vi "Get-module-path.vi"(8 "error in (no error)":errorcluster, 10 "Module type":T1=enum."Server", 11 "ModComm in":T2) -> (0 "error out":errorcluster, 2 "Module path":path, 3 "ModComm out":T2)   [LabVIEW 2013, in "SLMServer.lvlib" / "SLMServer.lvclass"]
uses:
  SLMServer.lvclass
  Object-reference.ctl
  Supported-module-types.ctl
  SLMServer.lvclass/SLMServer.ctl
  Read Max clients.vi
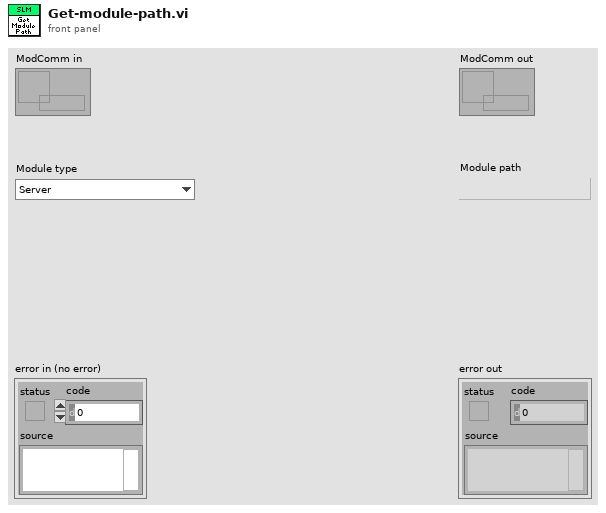
[diagram p1: front panel]
types:
  T1 = typedef "SLMServer.lvlib/SLMServer.lvclass/Supported-module-types.ctl" = enum16{"SLMControl", "PowderDeposition", "CameraVision", "Server", "All", "StrategyParser", "MaterialCharacterization", "StatusMonitor", "SLMSimulation", "LaserCharacterization"}
  T2 = typedef "SLMServer.lvlib/SLMServer.lvclass/Object-reference.ctl" = refnum<data-value>
  T3 = cluster{"Module type":T1, "MaxClients":i32, "Path":path, "Path type":bool}[]
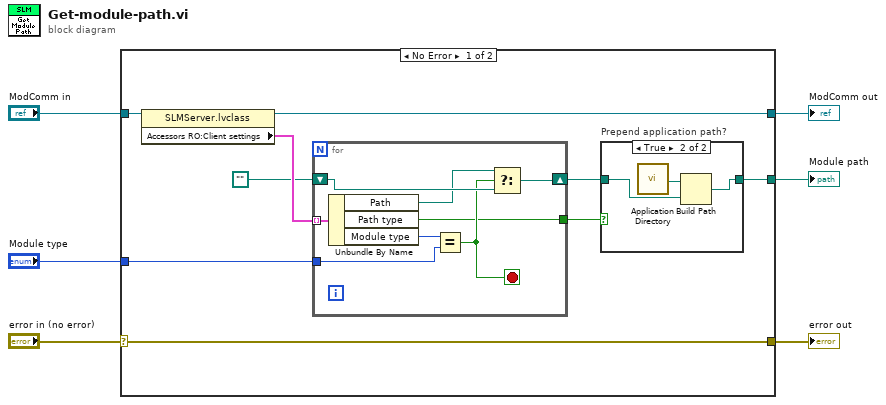
[diagram p0: block diagram]
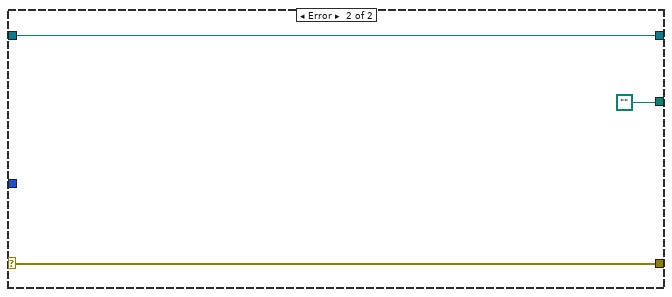
[diagram p3: hidden frame]
diagram:
  n1 = case shown="No Error" "error in (no error)" {
    selector: "error in (no error)" -> [w15 w30]
    tunnel: [w15 w30] -> w5
    tunnel: [w13 w29] -> w3
    tunnel: "ModComm in" -> [w14 w29]
    tunnel: "Module type" -> [w11 _]
    tunnel: [w7 path ""] -> w1
    frame No Error {
      n2 = property class="SLMServer.lvclass"(reference=w14) -> (reference out=w13:T2, "Accessors RO:Client settings"=w12:T3)  [unwired: 1 in, 1 out]
      n3 = for {
        tunnel: w12 -> [w27] mode=indexing
        tunnel: w11 -> [w26]
        shift-right: [w24] -> w9
        shift-left: path "" -> [w23]
        tunnel: [w20] -> w8
        stop <- w22 stop-if-true
        n4 = Unbundle By Name(w27) -> ("Path"=w21:path, "Path type"=w20:bool, "Module type"=w25:T1)
        n5 = Equal?(x=w25, y=w26) -> (x = y?=w22:bool)
        n6 = Select(t=w21, s=w22, f=w23) -> (s? t:f=w24:path)
      }
      n7 = case "Prepend application path?" shown="True" w8 {
        tunnel: w9 -> [w16 w19]
        tunnel: [w16 w17] -> w7
        frame False {
        }
        frame True {
          n8 = call <vilib>:"Application Directory.vi"() -> ("Application Directory"=w18:path)
          n9 = Build Path(base path=w18, name or relative path=w19) -> (appended path=w17:path)
        }
      }
    }
    frame Error {
    }
  }
  "error out" <- w5
  "ModComm out" <- w3
  "Module path" <- w1
